vi "example data for DUTLUG.vi"() -> (3 "linear data out":dbl[](array[numeric]))   [LabVIEW 2019]
panel:
  in  "linear":dbl[](array[numeric])=array[52067 elements]
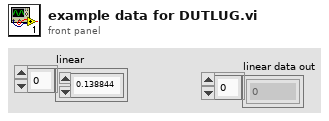
[diagram p1: front panel]
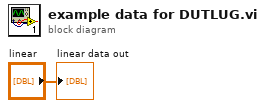
[diagram p0: block diagram]
diagram:
  "linear data out" <- "linear"
